vi "Port To Labels.vi"(8 "error in":errorcluster, 10 "direction":T1, 11 "port ref":T7 format="%.0x") -> (0 "error out":errorcluster, 2 "labels":T2[](array[typedef]), 3 "port ref out":T7 format="%.0x")   [LabVIEW 2020, in "Ballard ARINC 429 Scripting.lvlib"]
uses:
  Ballard ARINC 429 Scripting.lvlib
  <vilib>/NI VeriStand/Custom Device API/Custom Device Item Ref.ctl
  Shared/VS Channels Definition for Label.ctl
  Shared/VS Channel Definition for Parameter.ctl
  Shared/Direction.ctl
  Shared/Parameter Definition.ctl
  Encoding and Decoding/Encoding.ctl
  Shared/Transfer Type.ctl
  Encoding and Decoding/Encoding and Decoding.lvlib
  ARINC 429/ARINC 429 Scripting.lvlib
  <vilib>/NI VeriStand/Custom Device API/Custom Device API.lvlib
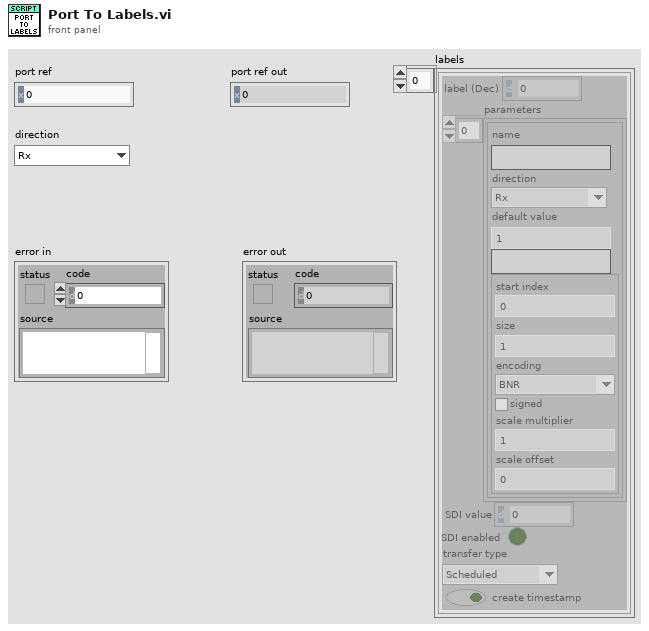
[diagram p1: front panel]
types:
  T1 = typedef "Direction.ctl" = enum16{"Rx", "Tx"}
  T2 = typedef "VS Channels Definition for Label.ctl" = cluster{"label (Dec)":u32, "parameters":T3[], "SDI value":u8, "SDI enabled":bool, "transfer type":T6, "create timestamp":bool}
  T3 = typedef "VS Channel Definition for Parameter.ctl" = cluster{"name":string, "direction":T1, "default value":dbl, "unit":string, "Parameter":T4}
  T4 = typedef "Parameter Definition.ctl" = cluster{"start index":i32, "size":i32, "encoding":T5, "signed":bool, "scale multiplier":dbl, "scale offset":dbl}
  T5 = typedef "Encoding and Decoding.lvlib/Encoding.ctl" = enum16{"BNR", "BCD", "Discrete"}
  T6 = typedef "Transfer Type.ctl" = enum16{"Scheduled", "Acyclic", "Block", "Strobe"}
  T7 = typedef "Custom Device API.lvlib/Custom Device Item Ref.ctl" = u64
  T8 = typedef "Label Properties.ctl" = cluster{"label (Dec)":T9, "SDI value":u8, "SDI enabled":bool}
  T9 = typedef "Label.ctl" = u8
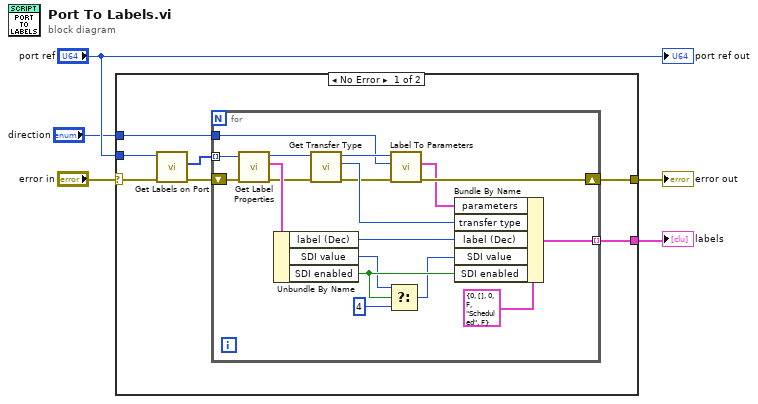
[diagram p0: block diagram]
diagram:
  n1 = case shown="No Error" "error in" {
    selector: "error in" -> [w7 w31]
    tunnel: "port ref" -> [w8 _]
    tunnel: [w11 w31] -> w5
    tunnel: [w12 _] -> w2
    tunnel: "direction" -> [w6 _]
    frame No Error {
      n2 = call "Get Labels on Port.vi"("error in"=w7, "port in"=w8) -> ("error out"=w10:errorcluster, "labels"=w9:T7[])  [unwired: 6 in, 2 out]
      n3 = for {
        tunnel: w9 -> [w29] mode=indexing
        tunnel: [w14] -> w12 mode=indexing
        shift-right: [w16] -> w11
        shift-left: w10 -> [w30]
        tunnel: w6 -> [w15]
        n4 = call "Get Label Properties.vi"("error in"=w30, "label ref in"=w29) -> ("error out"=w26:errorcluster, "label properties"=w27:T8, "label ref out"=w25:T7)  [unwired: 6 in, 1 out]
        n5 = Unbundle By Name(w27) -> ("label (Dec)"=w23:T9, "SDI value"=w21:u8, "SDI enabled"=w22:bool)
        n6 = call "Get Transfer Type.vi"("error in"=w26, "label ref in"=w25) -> ("error out"=w18:errorcluster, "transfer type"=w24:T6, "label ref out"=w17:T7)  [unwired: 7 in]
        n7 = Select(t=w21, s=w22, f=u8 4 ("SDI value")) -> (s? t:f=w19:u8)
        n8 = call "Label To Parameters.vi"("error in"=w18, "direction"=w15, "label ref"=w17) -> ("error out"=w16:errorcluster, "parameters"=w13:T3[])  [unwired: 6 in, 1 out]
        n9 = Bundle By Name(cluster=T2 {"label (Dec)"=0, "parameters"=[], "SDI value"=0, "SDI enabled"=FALSE, "transfer type"=enum."Scheduled", "create timestamp"=FALSE} ("label parameters"), "parameters"=w13, "transfer type"=w24, "label (Dec)"=w23, "SDI value"=w19, "SDI enabled"=w22) -> (w14:T2)
      }
    }
    frame Error {
    }
  }
  "error out" <- w5
  "labels" <- w2
  "port ref out" <- "port ref"
